vi "xcorr_packet ORIGINAL.vi"(0 "x":u32, 1 "y":u32, 2 "trigger":bool) -> (8 "out":u64, 9 "valid":bool)   [LabVIEW 2017]
uses:
  <vilib>/rvi/FXPMathLib/basic elements/FxpDiscreteDelay/XNode/nifxpmath_DiscreteDelay.xnode
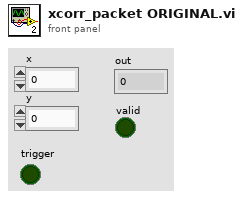
[diagram p1: front panel]
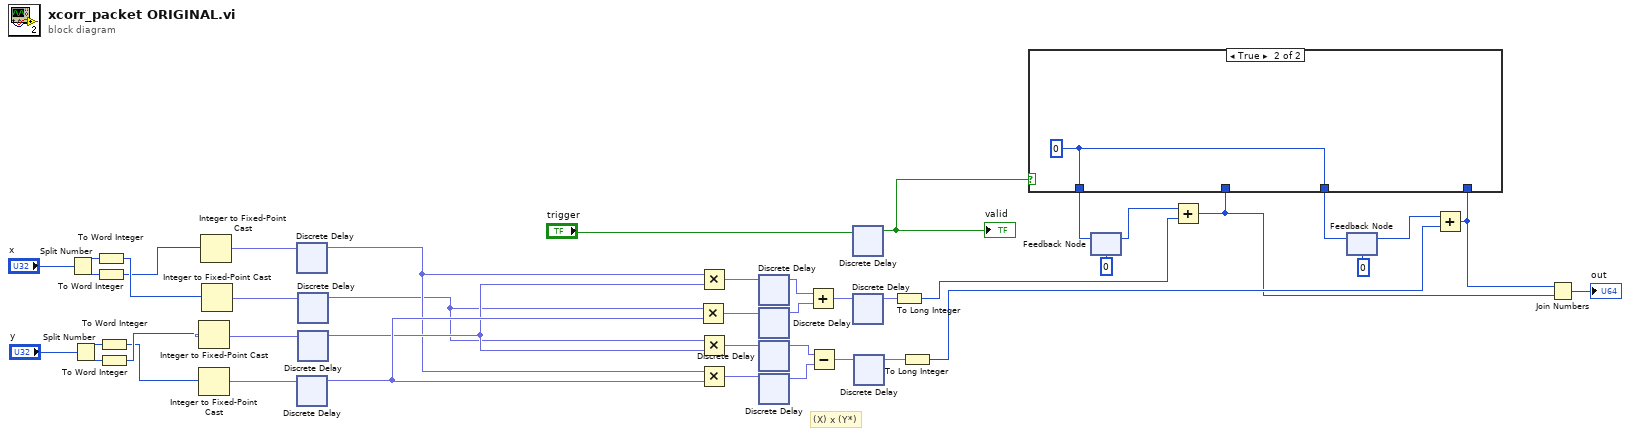
[diagram p0: block diagram]
diagram:
  # "(X) x (Y*)"
  n1 = Split Number(x="x") -> (hi(x)=w34:u16, lo(x)=w35:u16)
  n2 = Split Number(x="y") -> (hi(x)=w36:u16, lo(x)=w37:u16)
  n3 = To Word Integer(number=w34) -> (16bit integer=w8:i16)
  n4 = To Word Integer(number=w35) -> (16bit integer=w7:i16)
  n5 = To Word Integer(number=w36) -> (16bit integer=w5:i16)
  n6 = To Word Integer(number=w37) -> (16bit integer=w6:i16)
  n7 = Integer to Fixed-Point Cast(integer=w6) -> (fixed-point=w17:fxp<+/-,16,16>)  [unwired: 1 in]
  n8 = Integer to Fixed-Point Cast(integer=w5) -> (fixed-point=w19:fxp<+/-,16,16>)  [unwired: 1 in]
  n9 = Integer to Fixed-Point Cast(integer=w7) -> (fixed-point=w15:fxp<+/-,16,16>)  [unwired: 1 in]
  n10 = Integer to Fixed-Point Cast(integer=w8) -> (fixed-point=w16:fxp<+/-,16,16>)  [unwired: 1 in]
  n11 = xnode "Discrete Delay"("D"=w15) -> ("Q"=w4:fxp<+/-,16,16>)
  n12 = xnode "Discrete Delay"("D"=w19) -> ("Q"=w18:fxp<+/-,16,16>)
  n13 = xnode "Discrete Delay"("D"=w16) -> ("Q"=w3:fxp<+/-,16,16>)
  n14 = xnode "Discrete Delay"("D"=w17) -> ("Q"=w13:fxp<+/-,16,16>)
  n15 = Multiply(x=w3, y=w18) -> (x*y=w25:fxp<+/-,32,32>)
  n16 = Multiply(x=w4, y=w13) -> (x*y=w24:fxp<+/-,32,32>)
  n17 = Multiply(x=w3, y=w13) -> (x*y=w26:fxp<+/-,32,32>)
  n18 = Multiply(x=w4, y=w18) -> (x*y=w27:fxp<+/-,32,32>)
  n19 = xnode "Discrete Delay"("D"=w24) -> ("Q"=w20:fxp<+/-,32,32>)
  n20 = xnode "Discrete Delay"("D"=w25) -> ("Q"=w21:fxp<+/-,32,32>)
  n21 = xnode "Discrete Delay"("D"=w26) -> ("Q"=w22:fxp<+/-,32,32>)
  n22 = xnode "Discrete Delay"("D"=w27) -> ("Q"=w23:fxp<+/-,32,32>)
  n23 = Add(x=w20, y=w21) -> (x+y=w30:fxp<+/-,33,33>)
  n24 = Subtract(x=w22, y=w23) -> (x-y=w29:fxp<+/-,32,32>)
  n25 = xnode "Discrete Delay"("D"="trigger") -> ("Q"=w31:bool)
  "valid" <- w31
  n26 = xnode "Discrete Delay"("D"=w30) -> ("Q"=w14:fxp<+/-,33,33>)
  n27 = xnode "Discrete Delay"("D"=w29) -> ("Q"=w28:fxp<+/-,32,32>)
  n28 = To Long Integer(number=w14) -> (32bit integer=w32:i32)
  n29 = To Long Integer(number=w28) -> (32bit integer=w33:i32)
  n30 = feedback #1(0) -> (w40:i32)
  n31 = Add(x=w40, y=w32) -> (x+y=w1:i32)
  n32 = feedback #2(0) -> (w10:i32)
  n33 = Add(x=w10, y=w33) -> (x+y=w2:i32)
  n34 = case shown="True" w31 {
    tunnel: [w45 w46] -> w11
    tunnel: [w44 w46] -> w9
    tunnel: w1 -> [w44 _]
    tunnel: w2 -> [w45 _]
    frame False {
    }
    frame True {
      w46 = 0
    }
  }
  n35 = feedback-in #1(w9) -> ()
  n36 = feedback-in #2(w11) -> ()
  n37 = Join Numbers(hi=w2, lo=w1) -> ((hi.lo)=→"out":u64)
